vi "HatchAfterDriveAtDistance.vi"() -> ()   [LabVIEW 2018]
uses:
  Framework/Robot Global Data.vi
panel:
  in  "Collapse":bool
  in  "NoWait":bool
  in  "DistanceFromEnd":dbl
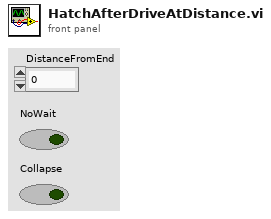
[diagram p1: front panel]
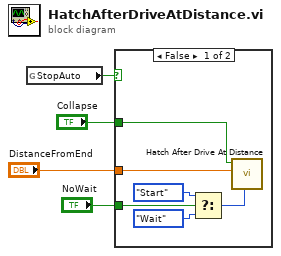
[diagram p0: block diagram]
diagram:
  n1 = global read "Robot Global Data.vi" "StopAuto"() -> (w4:bool)
  n2 = case shown="False" w4 {
    tunnel: "DistanceFromEnd" -> [w6 _]
    tunnel: "NoWait" -> [w8 _]
    tunnel: "Collapse" -> [w5 _]
    frame False {
      n3 = Select(t=enum16{"Start", "Wait"}."Start" ("Synchronization"), s=w8, f=enum16{"Start", "Wait"}."Wait" ("Synchronization")) -> (s? t:f=w7:enum16{"Start", "Wait"})
      n4 = call "Hatch After Drive At Distance.vi"("Synchronization"=w7, "DistanceFromEnd"=w6, "Collapsed?"=w5) -> ()  [unwired: 8 in, 1 out]
    }
    frame True {
    }
  }
